vi "Encoder doble.vi"() -> ()   [LabVIEW 2017]
uses:
  <vilib>/MakerHub/LINX/LMH-LINX.lvlib
  <vilib>/MakerHub/LINX/Public/Utilities/Open Serial.vi
  <vilib>/MakerHub/LINX/Public/Peripherals/Digital/Digital Read 1 Chan.vi
panel:
  in  "DI Channel 1":u8
  in  "DI Channel 2":u8
  in  "Serial Port":refnum<visa-resource-name>="N/A"
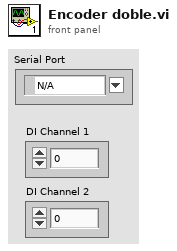
[diagram p1: front panel]
types:
  T1 = typedef "LMH-LINX.lvlib/LINX Ref.ctl" = cluster{"IO":T2, "Interface":T3, "LINX Device Config":T4}
  T2 = typedef "LMH-LINX.lvlib/Platform.ctl" = enum16{"Remote", "Local"}
  T3 = typedef "LMH-LINX.lvlib/Interface.ctl" = enum16{"Serial", "TCP"}
  T4 = typedef "LMH-LINX.lvlib/Device.lvlib/LINX Device Config.ctl" = cluster{"Interface":T3, "COM Port":refnum<visa-resource-name>, "TCP Configuration":T5, "Device Family":u8, "Device ID":u8, "Device Name":string, "TCP Ref":refnum<k5>, "Channels":T6}
  T5 = typedef "LMH-LINX.lvlib/Device.lvlib/TCP Config.ctl" = cluster{"IP Address":string, "Port":u16}
  T6 = typedef "LMH-LINX.lvlib/Channels.ctl" = cluster{"DI":u8[], "DO":u8[], "AI":u8[], "AO":u8[], "PWM":u8[], "QE":u8[], "UART":u8[], "I2C 2":u8[], "SPI":u8[], "CAN":u8[], "Servo":u8[], "AI Ref (V)":dbl, "AI Resolution (Bits)":u8, "AO Ref (V)":dbl, "AO Resolution (Bits)":u8}
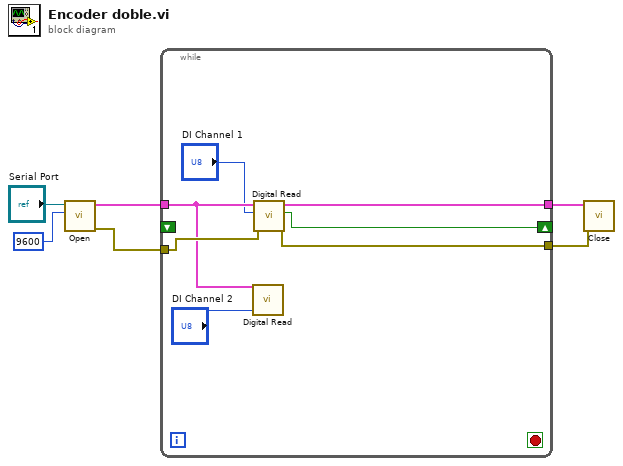
[diagram p0: block diagram]
diagram:
  n1 = call-poly <vilib>:"Open.vi"("Baud Rate Override"=u32 9600, "Serial Port"="Serial Port") -> ("Error Out"=w2:errorcluster, "LINX Resource"=w6:T1)  [unwired: 7 in, 1 out]
  n2 = while {
    tunnel: w6 -> [w9]
    tunnel: [w13] -> w5
    shift-right: [w12] -> _
    shift-left: _ -> [_]
    tunnel: w2 -> [w11]
    tunnel: [w10] -> w1
    stop <- _ stop-if-true
    n3 = call-poly <vilib>:"Digital Read.vi"("DI Channel"="DI Channel 2", "LINX Resource"=w9) -> ()  [unwired: 7 in, 3 out]
    n4 = call-poly <vilib>:"Digital Read.vi"("Error In"=w11, "DI Channel"="DI Channel 1", "LINX Resource"=w9) -> ("Error Out"=w10:errorcluster, "DI Value"=w12:bool, "LINX Resource"=w13:T1)  [unwired: 6 in]
  }
  n5 = call <vilib>:"Close.vi"("Error In"=w1, "LINX Resource"=w5) -> ()  [unwired: 9 in, 1 out]
